vi "XNET Database Add Alias.vi"(1 "default baud rate (0)":u64, 2 "default FD baud rate (0)":u64, 3 "CAN FD ISO mode (ISO)":u32(ring) items=["ISO", "Non ISO", "ISO Legacy"], 5 "alias":string, 7 "filepath":path, 11 "error in (no error)":errorcluster, 14 "ignore application protocol (F)":bool) -> (15 "error out":errorcluster)   [LabVIEW 2018]
doc: "Adds a new alias to a database file."
uses:
  nixlvapi.dll
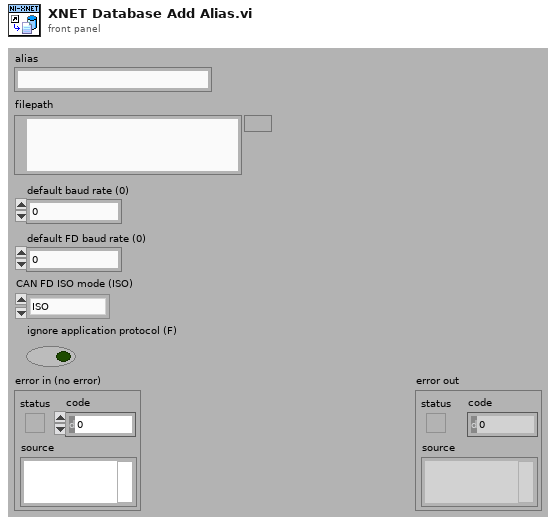
[diagram p1: front panel]
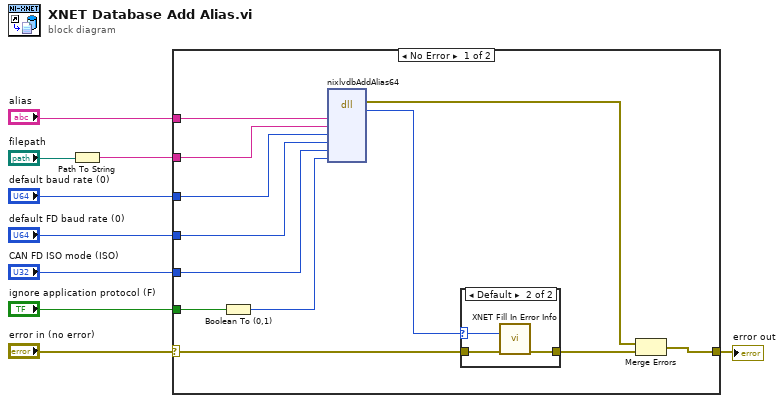
[diagram p0: block diagram]
diagram:
  n1 = Path To String(path="filepath") -> (string=w5:string)
  n2 = case shown="No Error" "error in (no error)" {
    selector: "error in (no error)" -> [w20 w26]
    tunnel: "alias" -> [w18 _]
    tunnel: [w11 w26] -> w9
    tunnel: w5 -> [w17 _]
    tunnel: "default baud rate (0)" -> [w16 _]
    tunnel: "default FD baud rate (0)" -> [w15 _]
    tunnel: "CAN FD ISO mode (ISO)" -> [w12 _]
    tunnel: "ignore application protocol (F)" -> [w14 _]
    frame No Error {
      n3 = Boolean To (0,1)(Boolean=w14) -> (0, 1=w13:i16)
      n4 = dll-call lib="nixlvapi.*" fn="nixlvdbAddAlias64" ("nilvxaiu.dll:lvxenDatabaseDeleteObject")("DatabaseAlias"=w18, "DatabaseFilepath"=w17, "DefaultBaudRate"=w16, "DefaultFDBaudRate"=w15, "DefaultCanFdIsoMode"=w12, "DefaultIgnApplProtocol"=w13) -> (error out=w10:errorcluster, "return type"=w19:i32)  [unwired: 9 in, 1 out]
      n5 = case shown="Default" w19 {
        selector: w19 -> [_ w23]
        tunnel: w20 -> [w22 w24]
        tunnel: [w22 w25] -> w21
        frame 0 {
        }
        frame Default {
          n6 = call "XNET Fill In Error Info.vi"("status code"=w23, "error in"=w24) -> ("error out"=w25:errorcluster)  [unwired: 13 out]
        }
      }
      n7 = Merge Errors(w10, w21) -> (w11:errorcluster)
    }
    frame Error {
    }
  }
  "error out" <- w9
